vi "Main.vi"() -> ()   [LabVIEW 2017, in "IteratorPatternDemo.lvclass"]
uses:
  IteratorPatternDemo.lvclass
  NameRepository Class/NameRepository.lvclass
  ConsoleOut/Print Options.ctl
  NameRepository Class/NameRepository.lvclass/NameRepository.ctl
  NameIterator Class/NameIterator.lvclass
panel:
  out "error out":errorcluster
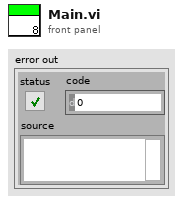
[diagram p1: front panel]
types:
  T1 = typedef "Print Options.ctl" = enum16{"Create", "Get Reference", "Print", "Print Header", "Close"}
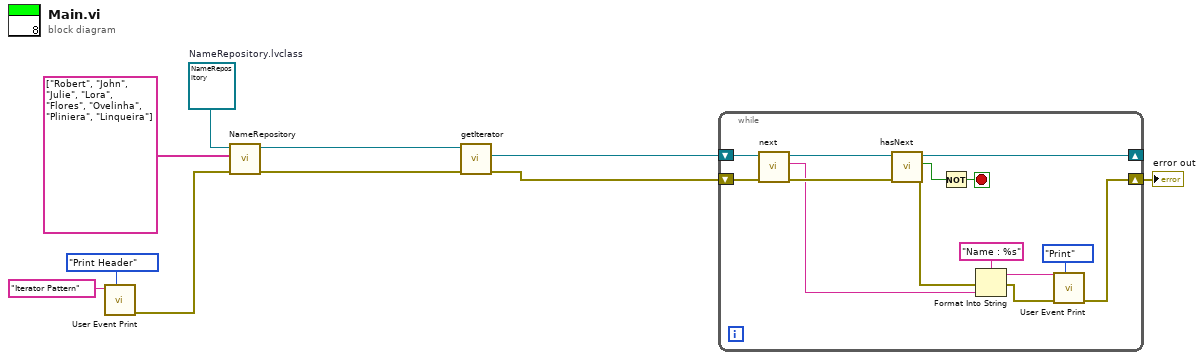
[diagram p0: block diagram]
diagram:
  w7 = refnum<class "NameRepository.lvclass"> refnum  # NameRepository.lvclass
  n1 = call "User Event Print.vi"("Options"=Print_Options."Print Header", "String to Print"="Iterator Pattern") -> ("error out"=w3:errorcluster)  [unwired: 8 in, 1 out]
  n2 = call "NameRepository.vi"("error in (no error)"=w3, "Names"=string[] ["Robert", "John", "Julie", "Lora", "Flores", "Ovelinha", "Pliniera", "Linqueira"], "NameRepository in"=w7) -> ("error out"=w6:errorcluster, "NameRepository out"=w10:refnum<class "NameRepository.lvclass">)  [unwired: 7 in]
  n3 = call-dynamic "getIterator.vi"("error in (no error)"=w6, "NameRepository in"=w10) -> ("error out"=w5:errorcluster, "NameIterator.lvclass"=w9:refnum<class "NameIterator.lvclass">)  [unwired: 7 in, 1 out]
  n4 = while {
    shift-right: [w17] -> _
    shift-left: w9 -> [w24]
    shift-right: [w11] -> w1
    shift-left: w5 -> [w16]
    stop <- w18 stop-if-true
    n5 = call-dynamic "next.vi"("error in (no error)"=w16, "NameIterator in"=w24) -> ("error out"=w22:errorcluster, "Name"=w20:string, "NameIterator out"=w23:refnum<class "NameIterator.lvclass">)  [unwired: 7 in]
    n6 = call-dynamic "hasNext.vi"("error in (no error)"=w22, "NameIterator in"=w23) -> ("error out"=w13:errorcluster, "hasNext?"=w19:bool, "NameIterator out"=w17:refnum<class "NameIterator.lvclass">)  [unwired: 7 in]
    n7 = Not(x=w19) -> (.not. x?=w18:bool)
    n8 = Format Into String(format string="Name : %s", error in=w13, w20) -> (resulting string=w15:string, error out=w12:errorcluster)  [unwired: 1 in]
    n9 = call "User Event Print.vi"("Options"=Print_Options."Print", "error in (no error)"=w12, "String to Print"=w15) -> ("error out"=w11:errorcluster)  [unwired: 7 in, 1 out]
  }
  "error out" <- w1
